vi "RichToFlatcif_channelcore_DestroyFIFOInstanceResponse.vi"(5 "OutputClusterType":T1, 11 "InputCluster":T3) -> (3 "OutputCluster":T1)   [LabVIEW 2021, in "CIFCoreChannel_client.lvlib"]
uses:
  cif_channelcore_DestroyFIFOInstanceResponse.ctl
  cif_common_Status.ctl
  cif_channelcore_DestroyFIFOInstanceResponse_Flat.ctl
  cif_common_Status_Flat.ctl
  CIFCoreChannel_client.lvlib
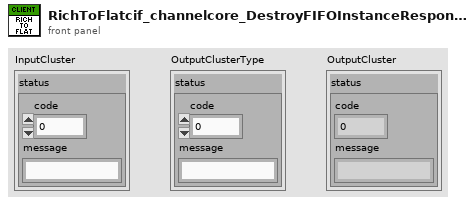
[diagram p1: front panel]
types:
  T1 = typedef "CIFCoreChannel_client.lvlib/cif_channelcore_DestroyFIFOInstanceResponse_Flat.ctl" = cluster{"status":T2}
  T2 = typedef "CIFCoreChannel_client.lvlib/cif_common_Status_Flat.ctl" = cluster{"code":i32, "message":string}
  T3 = typedef "CIFCoreChannel_client.lvlib/cif_channelcore_DestroyFIFOInstanceResponse.ctl" = cluster{"status":T4}
  T4 = typedef "CIFCoreChannel_client.lvlib/cif_common_Status.ctl" = cluster{"code":i32, "message":string}
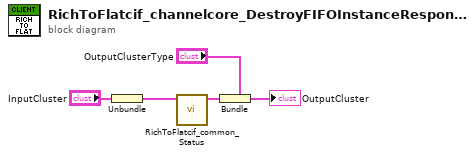
[diagram p0: block diagram]
diagram:
  n1 = Unbundle "Unbundle"("InputCluster") -> ("status"=w2:T4)
  n2 = call "RichToFlatcif_common_Status.vi"("InputCluster"=w2) -> ("OutputCluster"=w1:T2)  [unwired: 10 in]
  n3 = Bundle "Bundle"(cluster="OutputClusterType", "status"=w1) -> (→"OutputCluster":T1)
